vi "Get Name Index.vi"(0 "Display State In":T1, 5 "Current Name":string, 9 "Container State":T2, 11 "error in (no error)":errorcluster) -> (4 "Display State Out":T1, 6 "Name Index":i32, 15 "error out":errorcluster)   [LabVIEW 2011, in "X Listbox-Solution.xctl"]
doc: "This is an additional method that was added to the X Listbox to facilitate integration of the X Control into the Wind Turbine #2 VI. This VI is no longer used. To properly implement this feature, the user would need to modify the Display State event case and the X Listbox State.ctl\n\nAAL 9/09"
uses:
  X Listbox-Solution.xctl
  <vilib>/_xctls/Container State.ctl
  Abilities/X Listbox State.ctl
  <vilib>/_xctls/XControlSupport.lvlib
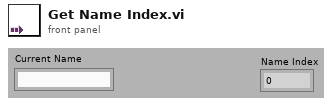
[diagram p1: front panel]
types:
  T1 = typedef "X Listbox-Solution.xctl/X Listbox State.ctl" = cluster{"# Items":i32, "Names":string[]}
  T2 = typedef "XControlSupport.lvlib/Container State.ctl" = cluster{"Indicator?":bool, "Run Mode?":bool, " Refnum":refnum<vi>}
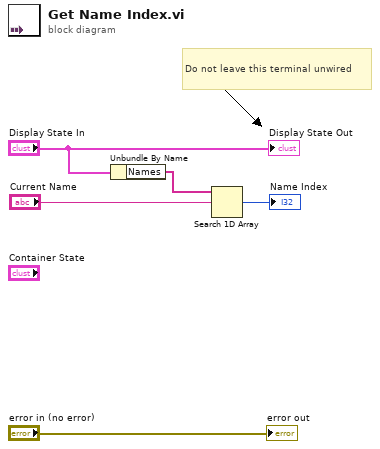
[diagram p0: block diagram]
diagram:
  # "Do not leave this terminal unwired"
  n1 = Unbundle By Name("Display State In") -> ("Names"=w2:string[])
  n2 = Search 1D Array(1D array=w2, element="Current Name") -> (index of element=→"Name Index":i32)  [unwired: 1 in]
  "Display State Out" <- "Display State In"
  "error out" <- "error in (no error)"
